vi "build matrix.vi"(11 "Current File Name":path) -> (2 "Real Matrix":T1, 3 "Dynamic Data":dynamicdata(waveform))   [LabVIEW 2011]
uses:
  <vilib>/Analysis/Matrix/Datatypes/RealMatrix.ctl
  <vilib>/Utility/file.llb/Read From Spreadsheet File (DBL).vi
  <vilib>/Analysis/Matrix/NI_Matrix.lvlib
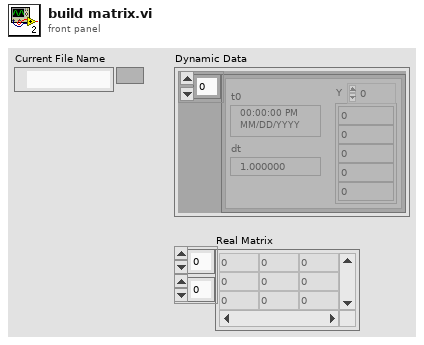
[diagram p1: front panel]
types:
  T1 = typedef "NI_Matrix.lvlib/RealMatrix.ctl" = dbl[][]
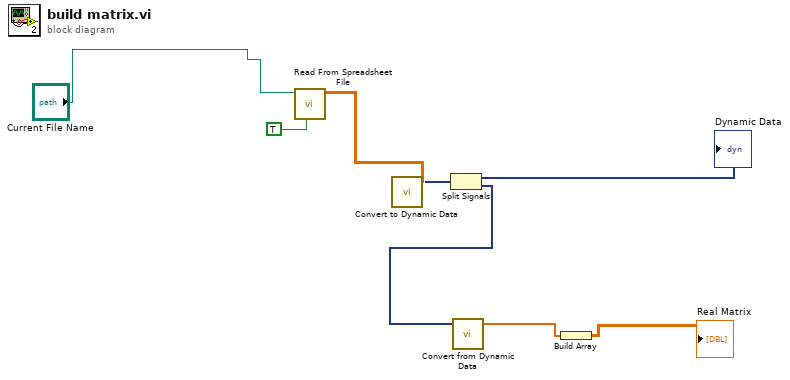
[diagram p0: block diagram]
diagram:
  n1 = call-poly <vilib>:"Read From Spreadsheet File.vi"("transpose (no:F)"=TRUE, "file path (dialog if empty)"="Current File Name") -> ("all rows"=w4:dbl[][])  [unwired: 5 in, 4 out]
  n2 = call "Convert to Dynamic Data"("2D Array"=w4) -> ("Dynamic Data Type"=w3:dynamicdata)  [unwired: 3 in]
  n3 = Split Signals(w3) -> (→"Dynamic Data":dynamicdata, w2:dynamicdata)  [unwired: 2 in]
  n4 = call "Convert from Dynamic Data"("Dynamic Data Type"=w2) -> ("Array"=w7:dbl[])  [unwired: 3 in]
  n5 = Build Array(w7) -> (→"Real Matrix":T1)
